vi "Main.vi"(0 "Wait_for_Popup":bool caption="Wait for Popup", 5 "Run_Popup":bool, 7 "Stop":bool) -> ()   [LabVIEW 2021]
doc: "This VI is the Main VI to run the Popup VI."
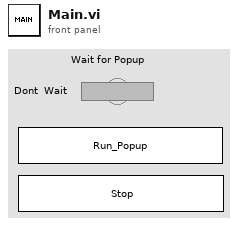
[diagram p1: front panel]
types:
  T1 = enum32{"Invalid", "Default", "Floating", "Floating/Auto-Hide", "Modal"}
  T2 = enum32{"Invalid", "Standard", "Closed", "Hidden", "Minimized", "Maximized"}
  T3 = enum32{"Bad", "Idle", "Run top level", "Running"}
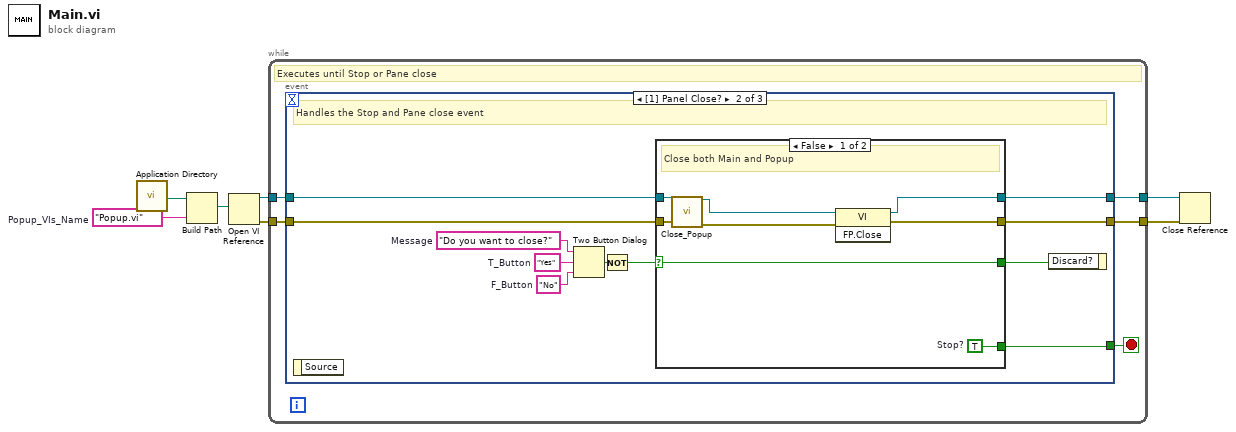
[diagram p0: block diagram]
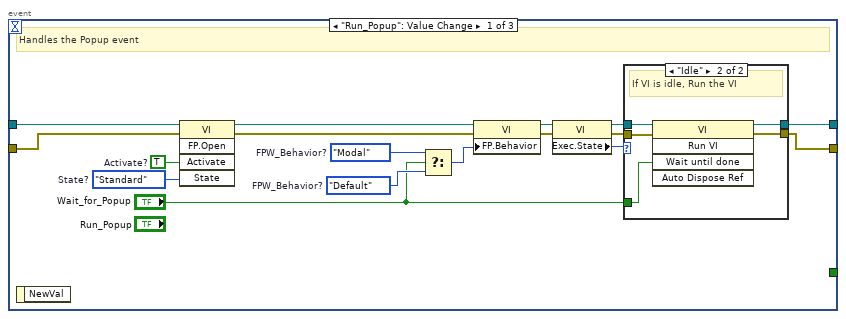
[diagram p2: hidden frame]
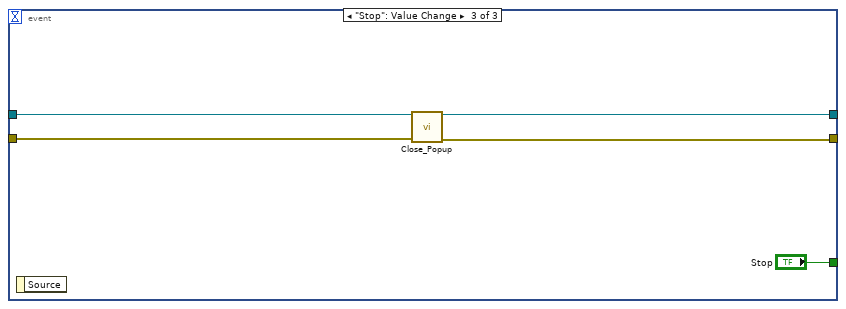
[diagram p5: hidden frame]
diagram:
  w2 = "Popup.vi"  # Popup_VIs_Name
  n1 = call <vilib>:"Application Directory.vi"() -> ("Application Directory"=w1:path)
  n2 = Build Path(base path=w1, name or relative path=w2) -> (appended path=w3:path)
  n3 = Open VI Reference(vi path=w3) -> (vi reference=w6:refnum<vi>, error out=w7:errorcluster)  [unwired: 5 in]
  n4 = while {
    tunnel: w7 -> [w11]
    tunnel: w6 -> [w10]
    tunnel: [w9] -> w5
    tunnel: [w8] -> w4
    stop <- w12 stop-if-true
    # "Executes until Stop or Pane close"
    n5 = event shown="[1] Panel Close?" {
      selector: _ -> [_ _ _]
      dyn-events: _ -> [_ _ _]
      timeout: _ -> [_ _ _]
      tunnel: [_ w37 "Stop"] -> w12
      tunnel: w11 -> [w27 w44 w62]
      tunnel: w10 -> [w26 w47 w63]
      tunnel: [w14 w45 w61] -> w9
      tunnel: [w13 w46 w60] -> w8
      event "Run_Popup": Value Change {
        w22 = T1."Modal"  # FPW_Behavior?
        w23 = T1."Default"  # FPW_Behavior?
        w28 = T2."Standard"  # State?
        w29 = TRUE  # Activate?
        # "Handles the Popup event"
        n6 = event-data() -> ()  [unwired: 1 in, 1 out]
        n7 = invoke on="Invoke Node" class="VI" method="FP.Open"(reference=w26, error in=w27, "Activate"=w29, "State"=w28) -> (reference out=w25:refnum<vi>, error out=w24:errorcluster)  [unwired: 1 in, 3 out]
        n8 = Select(t=w22, s="Wait_for_Popup", f=w23) -> (s? t:f=w20:T1)
        n9 = property on="Property Node" class="VI"(reference=w25, error in=w24, "FP.Behavior"=w20) -> (reference out=w19:refnum<vi>, error out=w16:errorcluster)
        n10 = property on="Property Node" class="VI"(reference=w19, error in=w16) -> (reference out=w18:refnum<vi>, error out=w17:errorcluster, "Exec.State"=w15:T3)
        n11 = case shown="\"Idle\"" w15 {
          tunnel: "Wait_for_Popup" -> [_ w36]
          tunnel: w18 -> [w31 w35]
          tunnel: w17 -> [w30 w34]
          tunnel: [w31 w33] -> w13
          tunnel: [w30 w32] -> w14
          frame Default {
            # "If the VI is running,\nDont Run it again"
          }
          frame "Idle" {
            # "If VI is idle, Run the VI"
            n12 = invoke on="Invoke Node" class="VI" method="Run VI"(reference=w35, error in=w34, "Wait until done"=w36) -> (reference out=w33:refnum<vi>, error out=w32:errorcluster)  [unwired: 2 in, 3 out]
          }
        }
      }
      event Panel Close? {
        w41 = "Do you want to close?"  # Message
        w42 = "Yes"  # T_Button
        w43 = "No"  # F_Button
        # "Handles the Stop and Pane close event"
        n13 = event-data() -> ()  [unwired: 1 in, 1 out]
        n14 = Two Button Dialog(message=w41, 1:w43, 2:w42) -> (T button?=w40:bool)
        n15 = Not(x=w40) -> (.not. x?=w38:bool)
        n16 = case shown="False" w38 {
          selector: w38 -> [w49 w58]
          tunnel: w47 -> [w55 w57]
          tunnel: [w53 w57] -> w46
          tunnel: [w51 w56] -> w45
          tunnel: w44 -> [w50 w56]
          tunnel: [w49 w58] -> w39
          tunnel: [w48 _] -> w37
          frame False {
            w48 = TRUE  # Stop?
            # "Close both Main and Popup"
            n17 = call "Close_Popup.vi"("Reference_In"=w55, "Error_In"=w50) -> ("Reference_Out"=w54:refnum<vi>, "Error_Out"=w52:errorcluster)  [unwired: 12 in]
            n18 = invoke on="Invoke Node" class="VI" method="FP.Close"(reference=w54, error in=w52) -> (reference out=w53:refnum<vi>, error out=w51:errorcluster)  [unwired: 1 in, 1 out]
          }
          frame True {
            # "Discard the pane close"
          }
        }
        n19 = event-data ("Event Filter Node")("Discard?"=w39) -> ()  [unwired: 1 in, 1 out]
      }
      event "Stop": Value Change {
        n20 = event-data() -> ()  [unwired: 1 in, 1 out]
        n21 = call "Close_Popup.vi"("Reference_In"=w63, "Error_In"=w62) -> ("Reference_Out"=w60:refnum<vi>, "Error_Out"=w61:errorcluster)  [unwired: 12 in]
      }
    }
  }
  n22 = Close Reference(reference=w4, error in (no error)=w5) -> ()  [unwired: 1 out]
